vi "Move From Double Click.vi"(8 "error in (no error)":errorcluster, 9 "Y (px)":i32, 10 "X (px)":i32, 11 "Stage Controller in":refnum<class "Stage Controller.lvclass">) -> (0 "error out":errorcluster, 3 "Stage Controller out":refnum<class "Stage Controller.lvclass">)   [LabVIEW 2023, in "Stage Controller.lvlib" / "Stage Controller.lvclass"]
uses:
  Stage Controller.lvclass
  Stage Controller.lvclass/Stage Controller.ctl
  Stage Axis.ctl
panel:
  out "Y out (mm)":dbl
  out "X out (mm)":dbl
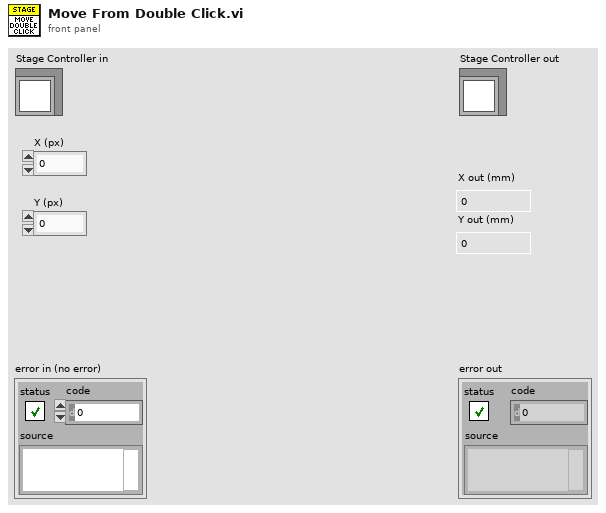
[diagram p1: front panel]
types:
  T1 = typedef "Stage Controller.lvlib/Stage Controller.lvclass/Stage Axis.ctl" = enum16{"unspecified", "X", "Y", "Z"}
  T2 = enum16{"Disabled", "ESP301", "Ti2", "Ludl", "ASI", "Simulate"}
  T3 = cluster{"top":dbl, "right":dbl, "width":dbl, "height":dbl}
  T4 = cluster{"Y Min":dbl, "Y Max":dbl, "X Min":dbl, "X Max":dbl}
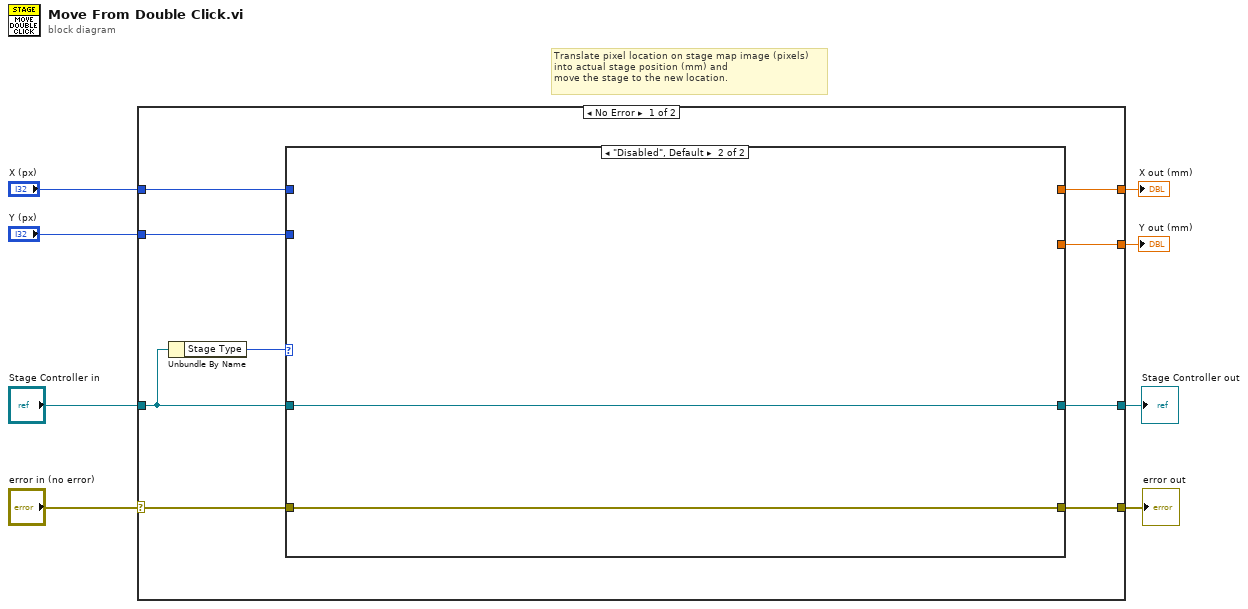
[diagram p0: block diagram]
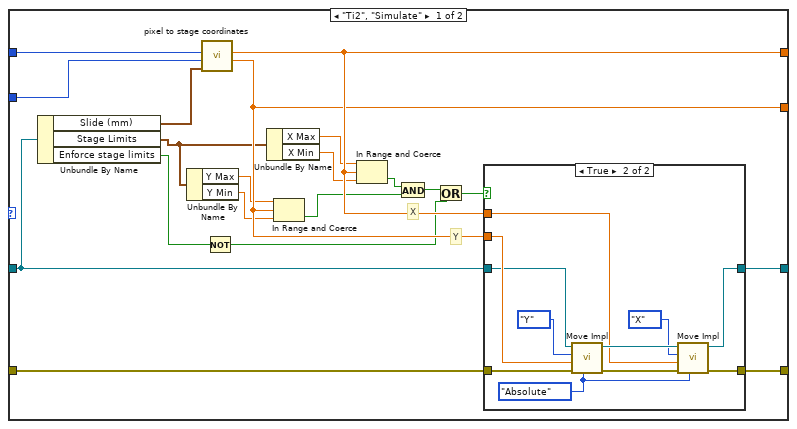
[diagram p2: hidden frame]
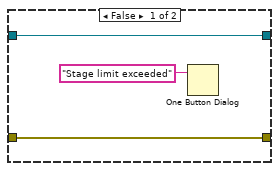
[diagram p3: hidden frame]
diagram:
  # "Translate pixel location on stage map image (pixels)\ninto actual stage position (mm) and\nmove the stage to the new location."
  n1 = case shown="No Error" "error in (no error)" {
    selector: "error in (no error)" -> [w12 w57]
    tunnel: [w11 w57] -> w7
    tunnel: [w17 w56] -> w5
    tunnel: "Stage Controller in" -> [w10 w56]
    tunnel: "X (px)" -> [w16 w55]
    tunnel: "Y (px)" -> [w15 w54]
    tunnel: [w14 w55] -> w2
    tunnel: [w13 w54] -> w1
    frame No Error {
      n2 = Unbundle By Name(w10) -> ("Stage Type"=w9:T2)
      n3 = case shown="\"Disabled\", Default" w9 {
        tunnel: [w37 w53] -> w17
        tunnel: w16 -> [w36 _]
        tunnel: w15 -> [w35 _]
        tunnel: [w34 _] -> w14
        tunnel: [w33 _] -> w13
        tunnel: w12 -> [w32 w52]
        tunnel: w10 -> [w31 w53]
        tunnel: [w18 w52] -> w11
        frame "Ti2", "Simulate" {
          # "Y"
          # "X"
          n4 = Unbundle By Name(w31) -> ("Slide (mm)"=w30:T3, "Stage Limits"=w19:T4, "Enforce stage limits"=w21:bool)
          n5 = Unbundle By Name(w19) -> ("Y Max"=w27:dbl, "Y Min"=w26:dbl)
          n6 = call "pixel to stage coordinates.vi"("Slide (mm)"=w30, "Y in (px)"=w35, "X in (px)"=w36) -> ("Y out (mm)"=w33:dbl, "X out (mm)"=w34:dbl)  [unwired: 7 in]
          n7 = Not(x=w21) -> (.not. x?=w20:bool)
          n8 = Unbundle By Name(w19) -> ("X Max"=w29:dbl, "X Min"=w28:dbl)
          n9 = In Range and Coerce(upper limit=w27, x=w33, lower limit=w26) -> (In Range?=w24:bool)  [unwired: 1 out]
          n10 = In Range and Coerce(upper limit=w29, x=w34, lower limit=w28) -> (In Range?=w25:bool)  [unwired: 1 out]
          n11 = And(x=w25, y=w24) -> (x .and. y?=w22:bool)
          n12 = Or(x=w22, y=w20) -> (x .or. y?=w23:bool)
          n13 = case shown="True" w23 {
            tunnel: w32 -> [w40 w51]
            tunnel: [w40 w46] -> w18
            tunnel: w34 -> [_ w42]
            tunnel: w33 -> [_ w50]
            tunnel: w31 -> [w38 w48]
            tunnel: [w38 w44] -> w37
            frame False {
              n14 = One Button Dialog(message="Stage limit exceeded") -> ()  [unwired: 1 in, 1 out]
            }
            frame True {
              w41 = enum16{"Relative", "Absolute"}."Absolute" ("Mode")
              n15 = call-dynamic "Move Impl.vi"("Mode"=w41, "error in (no error)"=w51, "Value (mm)"=w50, "Axis"=Stage_Axis."Y", "Stage Controller in"=w48) -> ("error out"=w47:errorcluster, "Stage Controller out"=w45:refnum<class "Stage Controller.lvclass">)  [unwired: 5 in]
              n16 = call-dynamic "Move Impl.vi"("Mode"=w41, "error in (no error)"=w47, "Value (mm)"=w42, "Axis"=Stage_Axis."X", "Stage Controller in"=w45) -> ("error out"=w46:errorcluster, "Stage Controller out"=w44:refnum<class "Stage Controller.lvclass">)  [unwired: 5 in]
            }
          }
        }
        frame "Disabled", Default {
        }
      }
    }
    frame Error {
    }
  }
  "error out" <- w7
  "Stage Controller out" <- w5
  "X out (mm)" <- w2
  "Y out (mm)" <- w1
